vi "onDestroy.vi"(8 "error in (no error)":errorcluster, 11 "XYStage":refnum<class "XYStage.lvclass">) -> (0 "error out":errorcluster, 3 "XYStage out":refnum<class "XYStage.lvclass">)   [LabVIEW 2015, in "XYStage.lvclass"]
doc: "JKI State Machine Objects (SMO) 1.0.4.18\nJKI - JKI\nCopyright (c) 2016, JKI"
uses:
  XYStage.lvclass
  <vilib>/JKI/JKI SMO/SMO/SMO.lvclass
panel:
  # "For instructions on how to use the JKI State Machine Objects, examples and video tutorials, visit:\nhttp://jki.net/state-machine-objects/\n\nJKI State Machine Objects™\nhttp://jki.net/state-machine-objects/\nCopyright (C) 2005-2015, JKI <info@jki.net>\nALL RIGHTS RESERVED"
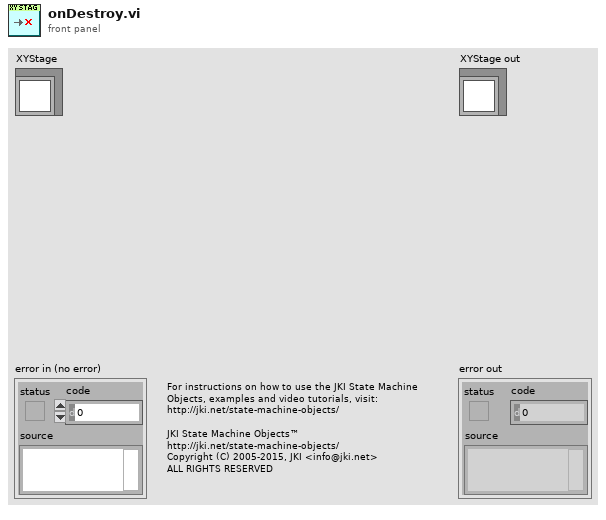
[diagram p1: front panel]
types:
  T1 = typedef "XYStage.lvclass/Dependencies--Cluster.ctl" = cluster{"Positions":refnum<class "SMO.Dictionary.Variant.lvclass">}
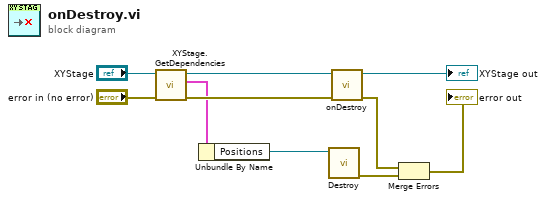
[diagram p0: block diagram]
diagram:
  n1 = call "XYStage.GetDependencies.vi"("error in (no error)"="error in (no error)", "XYStage"="XYStage") -> ("error out"=w6:errorcluster, "Dependencies"=w5:T1, "XYStage out"=w8:refnum<class "XYStage.lvclass">)  [unwired: 7 in]
  n2 = Unbundle By Name(w5) -> ("Positions"=w4:refnum<class "SMO.Dictionary.Variant.lvclass">)
  n3 = call <vilib>:"Destroy.vi"("SMO"=w4) -> ("error out"=w3:errorcluster)  [unwired: 10 in]
  n4 = call-parent "onDestroy.vi"("error in (no error)"=w6, "SMO"=w8) -> ("error out"=w2:errorcluster, "SMO out"=→"XYStage out":refnum<class "XYStage.lvclass">)  [unwired: 8 in]
  n5 = Merge Errors(w2, w3) -> (→"error out":errorcluster)
